vi "CRYWaveform to DAT.vi"(11 "Waveform In":T2={"Waveform"={"X0"=0.0, "dX"=0.0, "Y"=[]}, "X data"=1, "Y data"=0, "Y axis"=0, "X unit"="s", "Y unit"="", "Y dB ref"=1.0, "display Y"=TRUE, "display X"=FALSE, "Overload?"=FALSE, "Test Info"="", "Step No."=0, "Name"="", "protected"=FALSE, "Sqc history"=[], "Signal Channel ID"=0, "Plot Settings"={"Color"=0, "Interpolation"=0, "Point Style"=0, "Line Style"=0, "Point Color"=0, "Line Width"=0, "Bar Plot Style"=0, "Fill To"=0}, "AutoProtect"=FALSE} {"Y dB ref" format="%.1f"; "Y axis" items=["Log", "Lin"]; "Y data" items=["dB", "Lin"]; "X data" items=["dB", "Lin"]}) -> (3 "Curve Out":T1={"Name"="", "Curve"=[], "X data"=1, "Y data"=1, "Z data"=1, "X axis"=0, "Y axis"=1, "Z axis"=1, "X unit"="Hz", "Y unit"="", "Z unit"="deg.", "X dB ref"=1.0, "Y dB ref"=1.0, "Z dB ref"=1.0, "single val"=FALSE, "protected"=FALSE, "display X"=TRUE, "display Y"=TRUE, "display Z"=TRUE, "Test Info"="", "Step No."=0, "Plot Settings"={"Color"=0, "Interpolation"=0, "Point Style"=0, "Line Style"=0, "Point Color"=0, "Line Width"=0, "Bar Plot Style"=0, "Fill To"=0}, "AutoProtect"=FALSE} {"Z data" items=["dB", "Lin"]; "X data" items=["dB", "Lin"]; "Y data" items=["dB", "Lin"]; "Z dB ref" format="%.1f"; "Z axis" items=["Log", "Lin"]; "X dB ref" format="%.1f"; "X axis" items=["Log", "Lin"]; "Y axis" items=["Log", "Lin"]; "Y dB ref" format="%.1f"; "Curve"."z" format="%.2f"; "Curve"."y" format="%.2f"; "Curve"."x" format="%.2f"})   [LabVIEW 2013]
uses:
  Typedef Control/CRYWaveform Cluster.ctl
  Typedef Control/CRYData Cluster.ctl
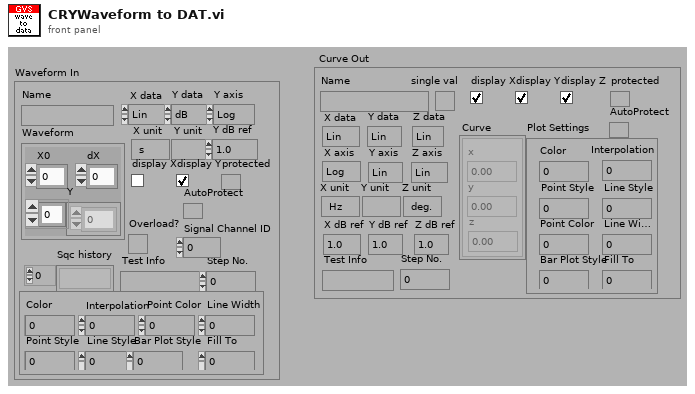
[diagram p1: front panel]
types:
  T1 = typedef "CRYData Cluster.ctl" = cluster{"Name":string, "Curve":cluster{"x":dbl, "y":dbl, "z":dbl}[], "X data":u16, "Y data":u16, "Z data":u16, "X axis":u16, "Y axis":u16, "Z axis":u16, "X unit":string, "Y unit":string, "Z unit":string, "X dB ref":dbl, "Y dB ref":dbl, "Z dB ref":dbl, "single val":bool, "protected":bool, "display X":bool, "display Y":bool, "display Z":bool, "Test Info":string, "Step No.":i32, "Plot Settings":cluster{"Color":u32, "Interpolation":u8, "Point Style":u8, "Line Style":u8, "Point Color":u32, "Line Width":u8, "Bar Plot Style":u8, "Fill To":i16}, "AutoProtect":bool}
  T2 = typedef "CRYWaveform Cluster.ctl" = cluster{"Waveform":cluster{"X0":dbl, "dX":dbl, "Y":sgl[]}, "X data":u16, "Y data":u16, "Y axis":u16, "X unit":string, "Y unit":string, "Y dB ref":dbl, "display Y":bool, "display X":bool, "Overload?":bool, "Test Info":string, "Step No.":i32, "Name":string, "protected":bool, "Sqc history":string[], "Signal Channel ID":i32, "Plot Settings":cluster{"Color":u32, "Interpolation":u8, "Point Style":u8, "Line Style":u8, "Point Color":u32, "Line Width":u8, "Bar Plot Style":u8, "Fill To":i16}, "AutoProtect":bool}
  T3 = cluster{"Color":u32, "Interpolation":u8, "Point Style":u8, "Line Style":u8, "Point Color":u32, "Line Width":u8, "Bar Plot Style":u8, "Fill To":i16}
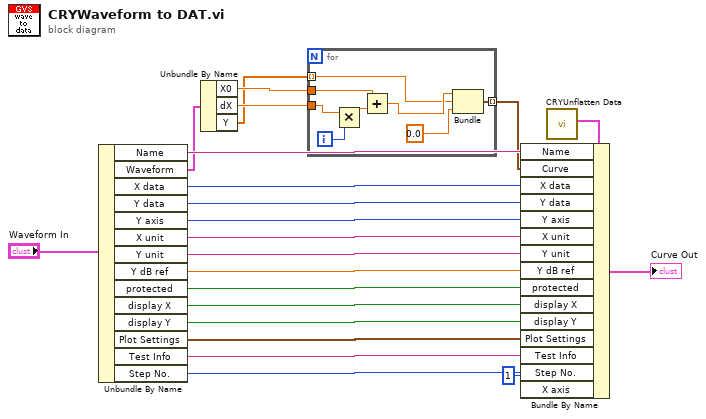
[diagram p0: block diagram]
diagram:
  n1 = Unbundle By Name("Waveform In") -> ("Name"=w21:string, "Waveform"=w20:cluster{"X0":dbl, "dX":dbl, "Y":sgl[]}, "X data"=w19:u16, "Y data"=w18:u16, "Y axis"=w17:u16, "X unit"=w16:string, "Y unit"=w15:string, "Y dB ref"=w14:dbl, "protected"=w12:bool, "display X"=w11:bool, "display Y"=w10:bool, "Plot Settings"=w9:T3, "Test Info"=w8:string, "Step No."=w3:i32)
  n2 = Unbundle By Name(w20) -> ("X0"=w6:dbl, "dX"=w7:dbl, "Y"=w4:sgl[])
  n3 = for {
    tunnel: w7 -> [w30]
    tunnel: w6 -> [w28]
    tunnel: [w26] -> w5 mode=indexing
    tunnel: w4 -> [w23] mode=indexing
    i -> [w24]
    n4 = Multiply(x=w30, y=w24) -> (x*y=w29:dbl)
    n5 = Add(x=w28, y=w29) -> (x+y=w25:dbl)
    n6 = Bundle(w25, "dt 2"=w23, "x+y"=0.0) -> (w26:cluster{dbl, "dt 2":sgl, "x+y":dbl})  [unwired: 1 out]
  }
  n7 = call "CRYUnflatten Data.vi"() -> ("Datum"=w2:T1)  [unwired: 9 in, 2 out]
  n8 = Bundle By Name(cluster=w2, "Name"=w21, "Curve"=w5, "X data"=w19, "Y data"=w18, "Y axis"=w17, "X unit"=w16, "Y unit"=w15, "Y dB ref"=w14, "protected"=w12, "display X"=w11, "display Y"=w10, "Plot Settings"=w9, "Test Info"=w8, "Step No."=w3, "X axis"=u16 1) -> (→"Curve Out":T1)
